vi "Rechnungsdaten2.vi"(8 "error in (no error)":errorcluster) -> (0 "error out":errorcluster)   [LabVIEW 2023]
uses:
  <vilib>/Utility/miscctls.llb/LVRectTypeDef.ctl
panel:
  in  "PLZ":dbl
  in  "Ort":string
  in  "Straße":string
  in  "Firmenname":string
  out "Firma":bool
  in  "Reserve Schalter 3":bool
  in  "Reserve Schalter 2":bool
  in  "Reserve Schalter":bool
  in  "Daten speichern":bool
  in  "Nachname":string
  in  "Vorname":string
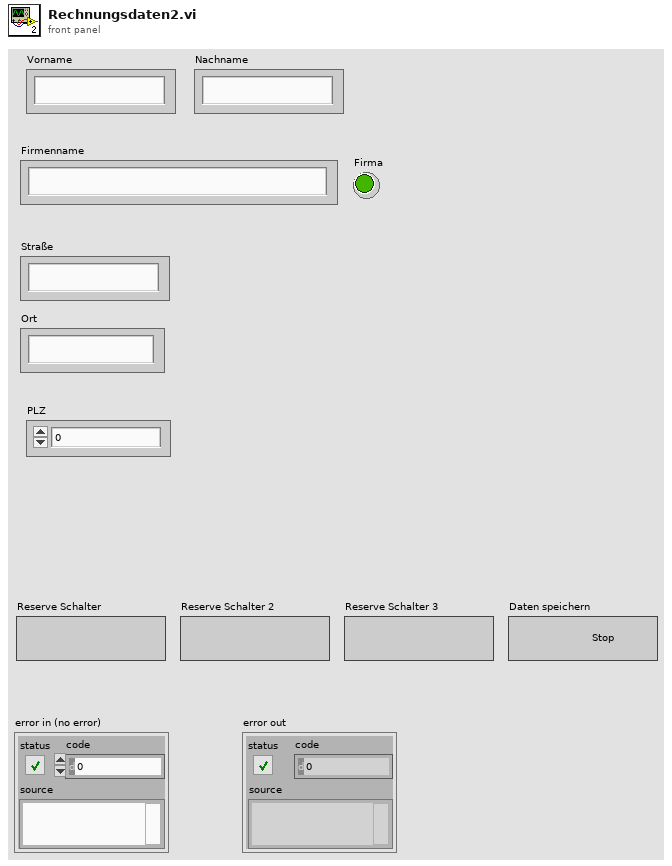
[diagram p1: front panel]
types:
  T1 = typedef "LVRectTypeDef.ctl" = cluster{"Left":i16, "Top":i16, "Right":i16, "Bottom":i16}
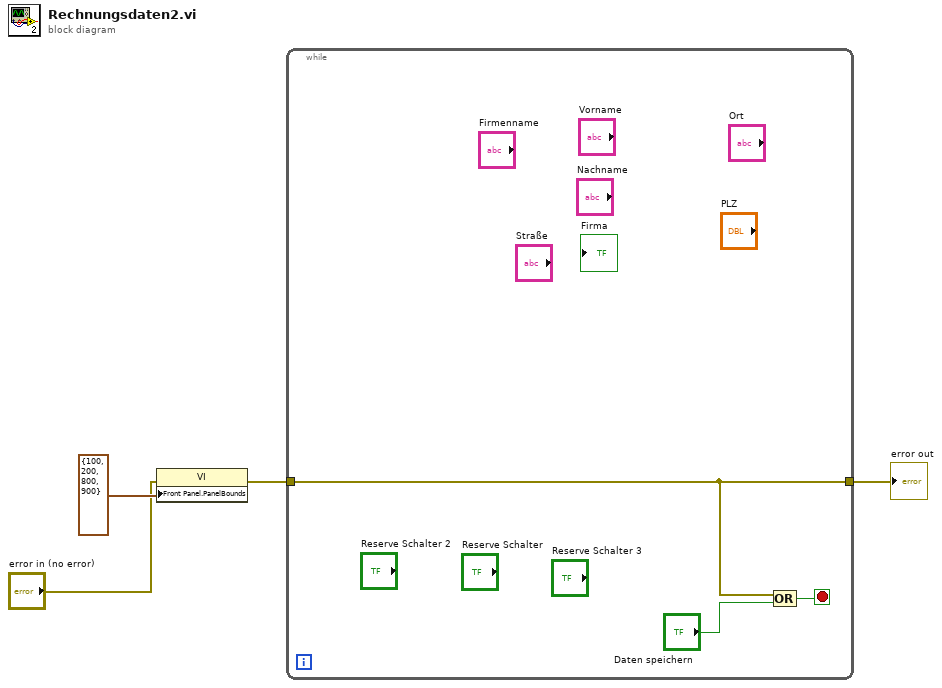
[diagram p0: block diagram]
diagram:
  n1 = property class="VI"(error in="error in (no error)", "Front Panel.PanelBounds"=T1 {"Left"=100, "Top"=200, "Right"=800, "Bottom"=900} ("Front Panel Window:Panel Bounds")) -> (error out=w1:errorcluster)  [unwired: 1 in, 1 out]
  n2 = while {
    tunnel: [w6] -> w4
    tunnel: w1 -> [w6]
    stop <- w5 stop-if-true
    n3 = Compound Arithmetic op=OR(w6, "Daten speichern") -> (w5:bool)
  }
  "error out" <- w4
